vi "Feature Step Name Chage.vi"() -> (1 "Feature Step Nameout":string, 3 "Next":bool)   [LabVIEW 2015]
panel:
  in  "Next":bool
  in  "stop":bool
  in  "Feature Step Name":string
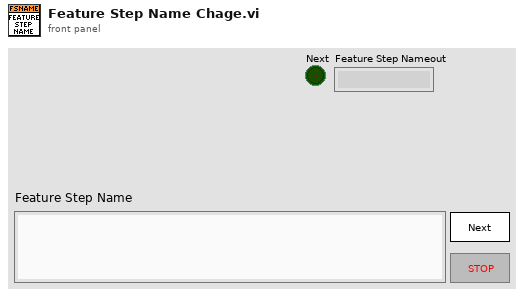
[diagram p1: front panel]
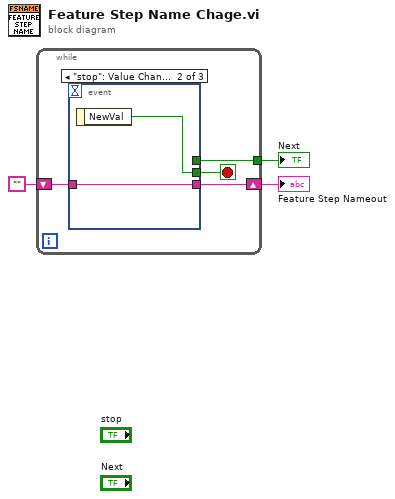
[diagram p0: block diagram]
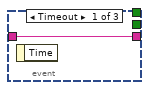
[diagram p2: hidden frame]
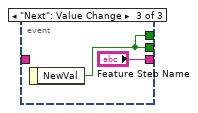
[diagram p3: hidden frame]
diagram:
  n1 = while {
    tunnel: [w6] -> w3
    shift-right: [w4] -> w2
    shift-left: "" -> [w5]
    stop <- w7 stop-if-true
    n2 = event shown="[1] \"stop\": Value Change" {
      selector: _ -> [_ _ _]
      dyn-events: _ -> [_ _ _]
      timeout: _ -> [_ _ _]
      tunnel: [_ w10 w12] -> w7
      tunnel: [_ _ w12] -> w6
      tunnel: [w8 w9 "Feature Step Name"] -> w4
      tunnel: w5 -> [w8 w9 _]
      event Timeout {
        n3 = event-data() -> ()  [unwired: 1 in, 1 out]
      }
      event "stop": Value Change {
        n4 = event-data() -> ("NewVal"=w10:bool)  [unwired: 1 in]
      }
      event "Next": Value Change {
        n5 = event-data() -> ("NewVal"=w12:bool)  [unwired: 1 in]
      }
    }
  }
  "Next" <- w3
  "Feature Step Nameout" <- w2
